vi "FileDialogCustom.vi"(8 "error in":errorcluster) -> (0 "error out":errorcluster, 2 "cancelled":bool, 3 "selected path":path)   [LabVIEW 2015]
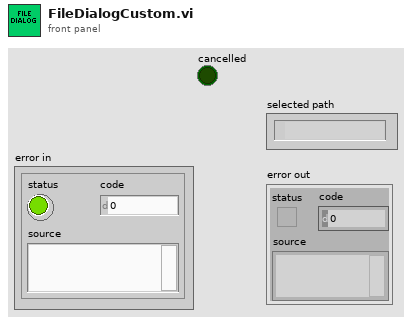
[diagram p1: front panel]
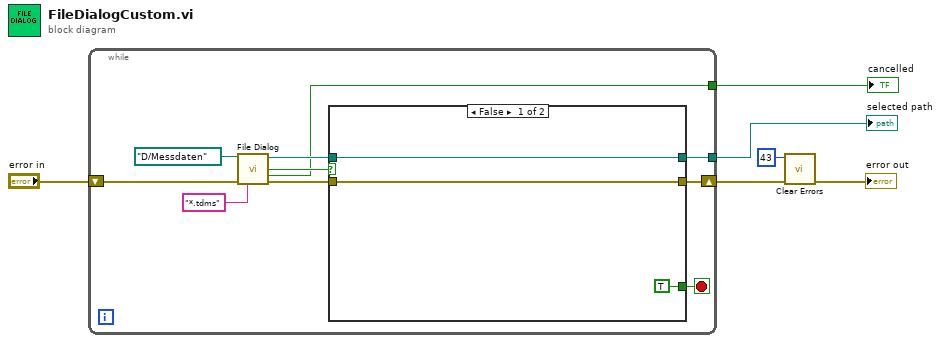
[diagram p0: block diagram]
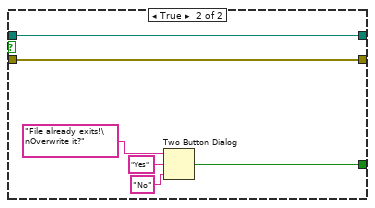
[diagram p2: hidden frame]
diagram:
  n1 = while {
    tunnel: [w13] -> w2
    shift-right: [w12] -> w6
    shift-left: "error in" -> [w16]
    tunnel: [w7] -> w1
    stop <- w10 stop-if-true
    n2 = call "File Dialog"("start path"=path "D:/Messdaten", "error in"=w16, "pattern (all files)"="*.tdms") -> ("selected path"=w14:path, "exists"=w15:bool, "cancelled"=w7:bool, "error out"=w11:errorcluster)  [unwired: 9 in]
    n3 = case shown="False" w15 {
      tunnel: w14 -> [w19 w20]
      tunnel: [w19 w20] -> w13
      tunnel: [w18 w21] -> w12
      tunnel: w11 -> [w18 w21]
      tunnel: [TRUE ("T button?") w22] -> w10
      frame False {
      }
      frame True {
        n4 = Two Button Dialog(message="File already exits!\nOverwrite it?", 1:"No" ("F button name (\"Cancel\")"), 2:"Yes" ("T button name (\"OK\")")) -> (T button?=w22:bool)
      }
    }
  }
  "selected path" <- w2
  "cancelled" <- w1
  n5 = call <vilib>:"Clear Errors.vi"("error in (no error)"=w6, "specific error code to clear (0: all)"=43) -> ("error out"=→"error out":errorcluster)  [unwired: 4 in, 1 out]
